vi "GUI_ManualParameterNumeric.vi"() -> ()   [LabVIEW 2013]
uses:
  Shared/GUI_Template/GUI_master/tcp_new_data_event.ctl
  Shared/GUI_Template/GUI_master/tcp new data cluster.ctl
panel:
  in  "value9::1":dbl caption="Value 9" min=-9999999.0 max=9999999.0
  in  "value8::1":dbl caption="Value 8" min=-9999999.0 max=9999999.0
  in  "value7::1":dbl caption="Value 7" min=-9999999.0 max=9999999.0
  in  "value6::1":dbl caption="Value 6" min=-9999999.0 max=9999999.0
  in  "value5::1":dbl caption="Value 5" min=-9999999.0 max=9999999.0
  in  "value4::1":dbl caption="Value 4" min=-9999999.0 max=9999999.0
  in  "value3::1":dbl caption="Value 3" min=-9999999.0 max=9999999.0
  in  "value2::1":dbl caption="Value 2" min=-9999999.0 max=9999999.0
  in  "value1::1":dbl caption="Value" min=-9999999.0 max=9999999.0
  in  "STOP":bool
  in  "restart":bool
  out "tcp data event":T1
  out "error IO 2":errorcluster
  in  "GUIdevice 1":string="ManualParameter_Lanex" caption="Device name"
  in  "insert tag":bool=TRUE
  # "Manual Parameter"
  # "to change device. just change name\nand press restart."
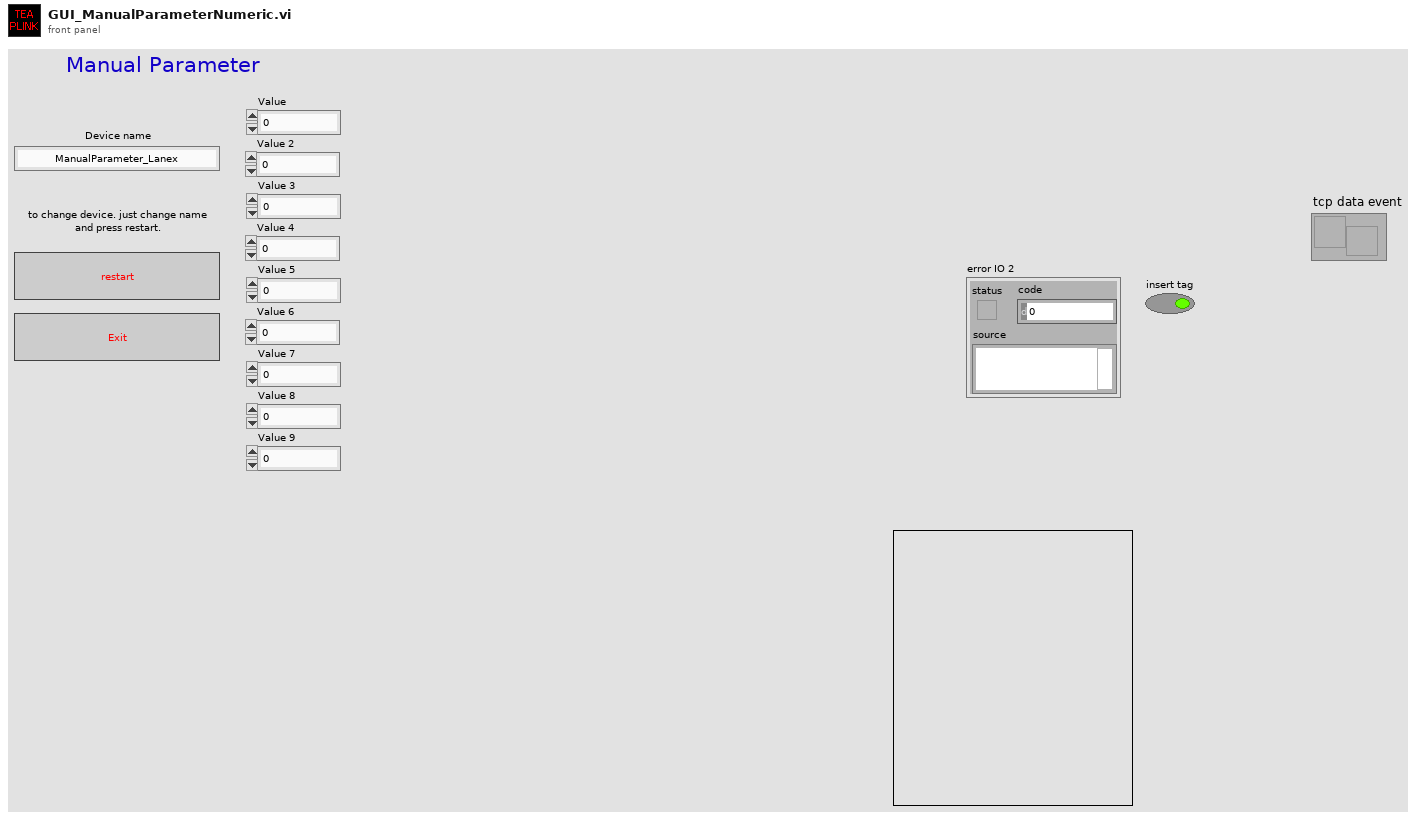
[diagram p1: front panel]
types:
  T1 = typedef "tcp_new_data_event.ctl" = refnum<user-event>
  T2 = typedef "tcp new data cluster.ctl" = cluster{"EventEnum":enum16{"new data", "connection status update"}, "Device name":string}
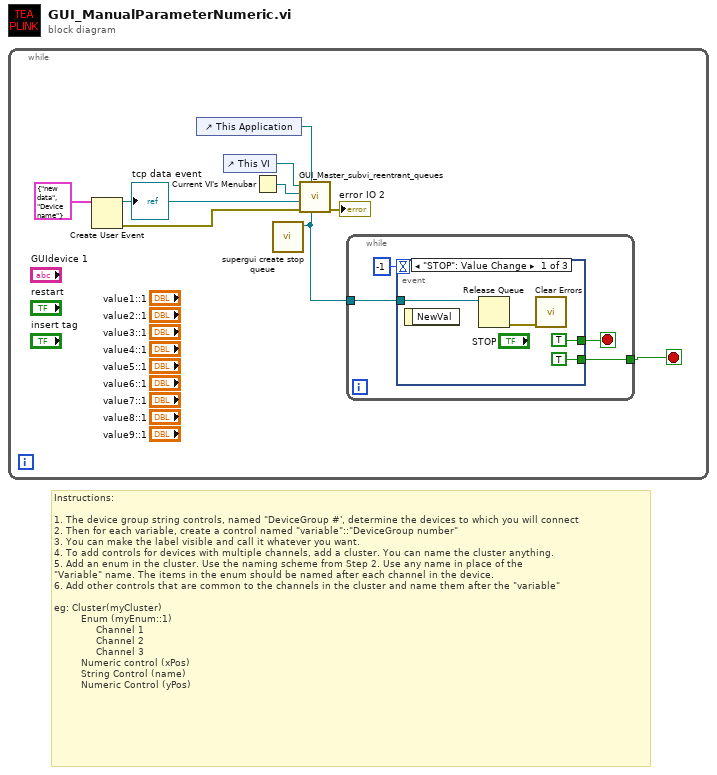
[diagram p0: block diagram]
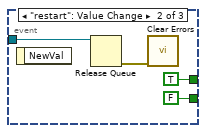
[diagram p2: hidden frame]
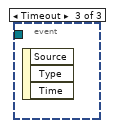
[diagram p3: hidden frame]
diagram:
  # "Instructions:\n\n1. The device group string controls, named \"DeviceGroup #', determine the devices to which you will connect\n2. Then for each variable, create a control named \"variable\"::\"DeviceGroup number\"\n3. You can make the label visible and call it whatever you want.\n4. To add controls for devices with multiple channels, add a cluster. You can name the cluster anything.\n5. Add an enum in the cluster. Use the naming scheme from Step 2. Use any name in place of the \n\"Variable\" name. The items in the enum should be named after each channel in the device. \n6. Add other controls that are common to the channels in the cluster and name them after the \"variable\"\n\neg: Cluster(myCluster)\n         Enum (myEnum::1)\n              Channel 1 \n              Channel 2\n              Channel 3\n         Numeric control (xPos)\n         String Control (name)\n         Numeric Control (yPos)"
  n1 = while {
    stop <- w1 stop-if-true
    n2 = Create User Event(user event datatype=T2 {"EventEnum"=enum."new data", "Device name"="Device name"} ("New Event")) -> (user event=w4:refnum<user-event>, error out=w5:errorcluster)  [unwired: 1 in]
    "tcp data event" <- w4
    n3 = control-ref of="This Application"() -> (w3:refnum<vi>)
    n4 = control-ref of="This VI"() -> (w8:refnum<vi>)
    n5 = Current VI's Menubar() -> (w7:refnum<k9>)
    n6 = call "supergui create stop queue.vi"() -> ("STOP Queue out"=w2:refnum<queue>)  [unwired: 11 in]
    n7 = call "GUI_Master_subvi_reentrant_queues.vi"("STOP Queue in"=w2, "This Application"=w3, "error in (no error)"=w5, "tcp data event"=w4, "Caller menu reference"=w7, "Caller VI ref"=w8) -> ("error out"=→"error IO 2":errorcluster)  [unwired: 5 in]
    n8 = while {
      tunnel: w2 -> [w11]
      tunnel: [w10] -> w1
      stop <- w12 stop-if-true
      n9 = event shown="[0] \"STOP\": Value Change" {
        selector: _ -> [_ _ _]
        dyn-events: _ -> [_ _ _]
        timeout: -1 -> [_ _ _]
        tunnel: [TRUE ("STOP") TRUE ("STOP") _] -> w12
        tunnel: w11 -> [w15 w19 _]
        tunnel: [TRUE ("STOP") FALSE ("STOP") _] -> w10
        event "STOP": Value Change {
          n10 = event-data() -> ()  [unwired: 1 in, 1 out]
          n11 = Release Queue(queue=w15) -> (error out=w16:errorcluster)  [unwired: 2 in, 2 out]
          n12 = call <vilib>:"Clear Errors.vi"("error in (no error)"=w16) -> ()  [unwired: 6 in, 1 out]
        }
        event "restart": Value Change {
          n13 = event-data() -> ()  [unwired: 1 in, 1 out]
          n14 = Release Queue(queue=w19) -> (error out=w20:errorcluster)  [unwired: 2 in, 2 out]
          n15 = call <vilib>:"Clear Errors.vi"("error in (no error)"=w20) -> ()  [unwired: 6 in, 1 out]
        }
        event Timeout {
          n16 = event-data() -> ()  [unwired: 1 in, 3 out]
        }
      }
    }
  }
